vi "CRYInsert VI into SubPanel.vi"(9 "options":i32, 10 "WindowType":string="DockState", 11 "SubPanel Ref":refnum<vi>) -> (0 "WindowName":string, 1 "Icon Out":string, 2 "VI Ref Out":refnum<vi>, 3 "SubPanel Ref Out":refnum<vi>)   [LabVIEW 2013]
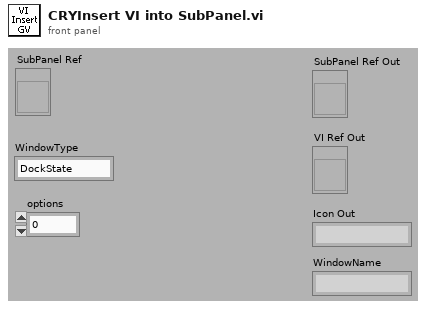
[diagram p1: front panel]
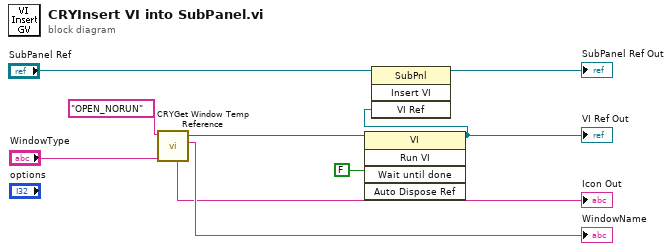
[diagram p0: block diagram]
diagram:
  n1 = call "CRYGet Window Temp Reference.vi"("sWindowName"="WindowType", "sAction"="OPEN_NORUN") -> ("sTitleName Out"=→"WindowName":string, "pVIRef_Out"=w8:refnum<vi>, "sIcon_Out"=→"Icon Out":string)  [unwired: 2 in, 5 out]
  n2 = invoke class="VI" method="Run VI"(reference=w8, "Wait until done"=FALSE ("Wait Until Done")) -> (reference out=w5:refnum<vi>)  [unwired: 3 in, 4 out]
  "VI Ref Out" <- w5
  n3 = invoke on="Invoke Node" class="SubPnl" method="Insert VI"(reference="SubPanel Ref", "VI Ref"=w5) -> (reference out=→"SubPanel Ref Out":refnum<vi>)  [unwired: 2 in, 3 out]
